vi "Nattify - Move All BD Objects.vi"(0 "VI in":refnum<vi>, 5 "x delta":i32, 7 "y delta":i32, 11 "error in":errorcluster) -> (15 "error out":errorcluster)   [LabVIEW 2020]
uses:
  <vilib>/Utility/miscctls.llb/LVDeltaXY32Cluster.ctl
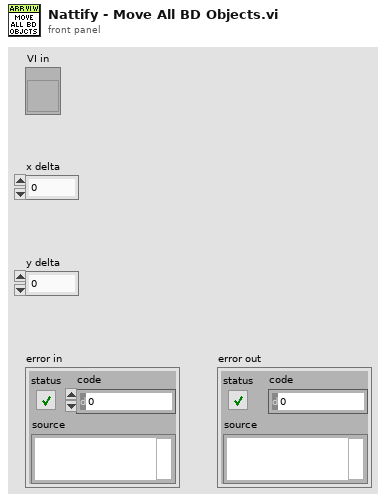
[diagram p1: front panel]
types:
  T1 = typedef "LVDeltaXY32Cluster.ctl" = cluster{"X":i32, "Y":i32}
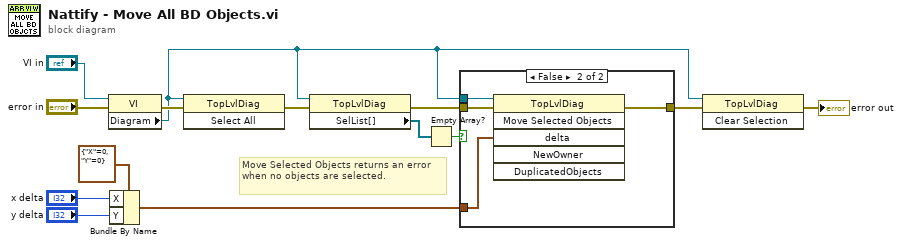
[diagram p0: block diagram]
diagram:
  # "Move Selected Objects returns an error when no objects are selected."
  n1 = property class="VI"(reference="VI in", error in="error in") -> (error out=w14:errorcluster, "Diagram"=w3:refnum<vi>)  [unwired: 1 out]
  n2 = Bundle By Name(cluster=T1 {"X"=0, "Y"=0} ("X/Y Delta"), "X"="x delta", "Y"="y delta") -> (w13:T1)
  n3 = invoke class="TopLvlDiag" method="Select All"(reference=w3, error in=w14) -> (error out=w5:errorcluster)  [unwired: 1 in, 2 out]
  n4 = property class="TopLvlDiag"(reference=w3, error in=w5) -> (error out=w4:errorcluster, "SelList[]"=w1:refnum<vi>[])  [unwired: 1 out]
  n5 = Empty Array?(array=w1) -> (empty?=w2:bool)
  n6 = case shown="False" w2 {
    tunnel: w13 -> [_ w19]
    tunnel: [w15 w18] -> w8
    tunnel: w4 -> [w15 w17]
    tunnel: w3 -> [_ w16]
    frame True {
    }
    frame False {
      n7 = invoke class="TopLvlDiag" method="Move Selected Objects"(reference=w16, error in=w17, "delta"=w19) -> (error out=w18:errorcluster)  [unwired: 3 in, 5 out]
    }
  }
  n8 = invoke class="TopLvlDiag" method="Clear Selection"(reference=w3, error in=w8) -> (error out=→"error out":errorcluster)  [unwired: 1 in, 2 out]
